vi "Becker-Hickl Read Single I32.vi"(8 "Error In":errorcluster, 10 "Default":i32, 11 "Bytes in":string) -> (0 "Error Out":errorcluster, 2 "I32":i32, 3 "Bytes out":string)   [LabVIEW 2021, in "Becker-Hickl Files.lvlib"]
uses:
  Becker-Hickl Files.lvlib
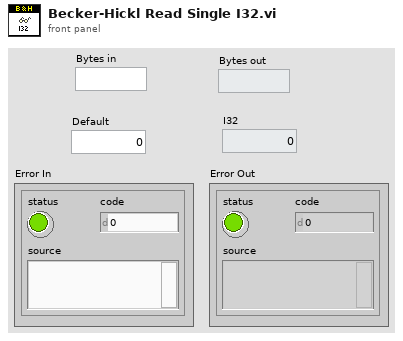
[diagram p1: front panel]
types:
  T1 = enum16{"big-endian, network order", "native, host order", "little-endian"}
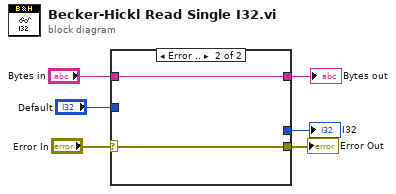
[diagram p0: block diagram]
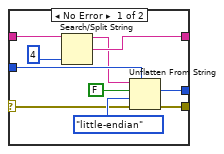
[diagram p2: hidden frame]
diagram:
  n1 = case shown="Error .." "Error In" {
    selector: "Error In" -> [w8 w17]
    tunnel: [w13 _] -> w6
    tunnel: [w14 w18] -> w5
    tunnel: "Bytes in" -> [w16 w18]
    tunnel: "Default" -> [w12 _]
    tunnel: [w7 w17] -> w1
    frame No Error {
      n2 = Search/Split String(string=w16, offset (0)=4 ("index")) -> (substring before match=w11:string, match + rest of string=w14:string)  [unwired: 1 in, 1 out]
      n3 = Unflatten From String(type=w12, binary string=w11, data includes array or string size? (T)=FALSE, byte order (0:big-endian, network order)=T1."little-endian", error in (no error)=w8) -> (value=w13:i32, error out=w7:errorcluster)  [unwired: 1 out]
    }
    frame Error {
    }
  }
  "I32" <- w6
  "Bytes out" <- w5
  "Error Out" <- w1
